vi "sample.vi"(8 "error in (no error)":errorcluster caption="entrée d'erreur (pas d'erreur)", 11 "Mixture.lvclass":refnum<class "Mixture.lvclass">) -> (0 "error out":errorcluster caption="sortie d'erreur", 2 "out":cluster{"X":dbl[][], "y":dbl[]}, 3 "Mixture.lvclass 2":refnum<class "Mixture.lvclass">)   [LabVIEW 2020, in "Mixture.lvclass"]
doc: "Generate random samples from the fitted Gaussian distribution."
uses:
  Mixture.lvclass
  C:/Users/cipop/TDF Dropbox/2_Technologies de France/1 - Services et Etudes/PLAIY/2 - DEV/PLAIYLAB/code/Python/Python.lvclass
  C:/Users/cipop/TDF Dropbox/2_Technologies de France/1 - Services et Etudes/PLAIY/2 - DEV/PLAIYLAB/code/Model/Model.lvclass
  Mixture.lvclass/Mixture.ctl
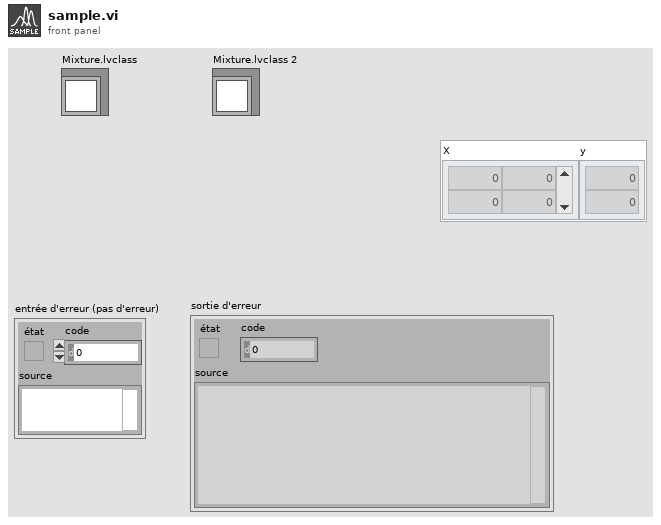
[diagram p1: front panel]
types:
  T1 = typedef "data.ctl" = cluster{"name":string, "X":dbl[][]}
  T2 = typedef "mixture_data.ctl" = cluster{"n_samples":dbl}
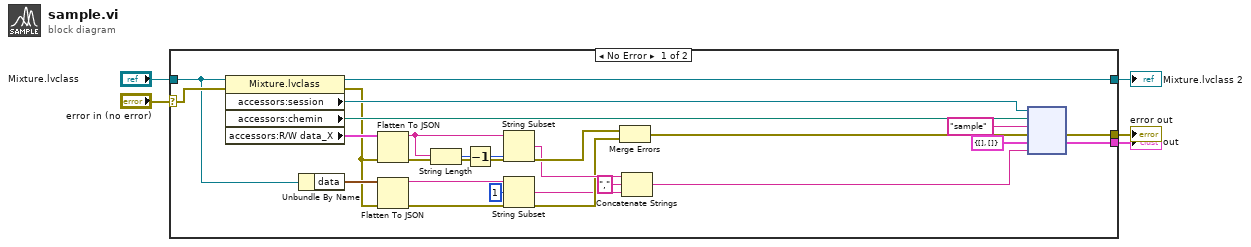
[diagram p0: block diagram]
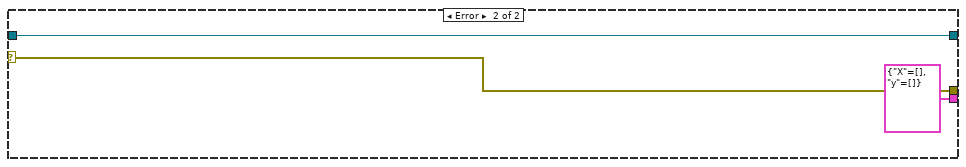
[diagram p2: hidden frame]
diagram:
  n1 = case shown="No Error" "error in (no error)" {
    selector: "error in (no error)" -> [w27 w32]
    tunnel: [w28 w32] -> w2
    tunnel: [w6 w31] -> w3
    tunnel: "Mixture.lvclass" -> [w12 w31]
    tunnel: [w14 cluster{"X":dbl[][], "y":dbl[]} {"X"=[], "y"=[]} ("out")] -> w1
    frame No Error {
      n2 = property class="Mixture.lvclass"(reference=w12, error in=w27) -> (reference out=w6:refnum<class "Mixture.lvclass">, error out=w8:errorcluster, "accessors:session"=w10:refnum<k35>, "accessors:chemin"=w9:path, "accessors:R/W data_X"=w13:T1)
      n3 = Unbundle By Name(w12) -> ("data"=w11:T2)
      n4 = Flatten To JSON(anything=w13, error in (no error)=w8) -> (JSON string=w24:string, 11:w21:errorcluster)  [unwired: 1 in]
      n5 = Flatten To JSON(anything=w11, error in (no error)=w8) -> (JSON string=w22:string, 11:w18:errorcluster)  [unwired: 1 in]
      n6 = String Length(string=w24) -> (length=w26:i32)
      n7 = Decrement(x=w26) -> (x-1=w25:i32)
      n8 = String Subset(string=w24, length (rest)=w25) -> (substring=w20:string)  [unwired: 1 in]
      n9 = String Subset(string=w22, offset (0)=1) -> (substring=w16:string)  [unwired: 1 in]
      n10 = Merge Errors(w21, w18) -> (w7:errorcluster)
      n11 = Concatenate Strings(w20, "," ("string"), w16) -> (w19:string)
      n12 = node(w10, w9, "sample" ("nom de la fonction"), w7, cluster{"X":dbl[][], "y":dbl[]} {"X"=[], "y"=[]} ("out"), w19) -> (w28:errorcluster, w14:cluster{"X":dbl[][], "y":dbl[]})  [unwired: 1 in, 3 out]
    }
    frame Error {
    }
  }
  "error out" <- w2
  "Mixture.lvclass 2" <- w3
  "out" <- w1
